vi "OnButton.vi"   [LabVIEW 2015]
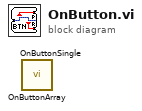
[diagram p0: block diagram]
diagram:
  n1 = call "OnButtonArray.vi"() -> ()  [unwired: 1 in, 2 out]
  n2 = call "OnButtonSingle.vi"() -> ()  [unwired: 1 in, 2 out]
